vi "Teleop.vi"(10 "Match Info":T1={"Autonomous Elapsed Seconds"=0.0, "TeleOp Elapsed Seconds"=0.0, "Disabled Elapsed Seconds"=0.0, "Visited Autonomous"=FALSE, "Visited TeleOp"=FALSE, "Visited Disabled"=FALSE, "Autonomous Settings"={"Autonomous Style"=enum."Independent", "VI Refnum"=refnum}}) -> ()   [LabVIEW 2017]
doc: "This VI is called for each TeleOp packet received from the DS where the robot is not disabled. It is often used to read from the joysticks and update I/O or to update setpoints for timed control loops. It should complete and return within 20 milliseconds or it may miss DS packets."
uses:
  <vilib>/Rock Robotics/WPI/DriverStation/WPI_DriverStationMatch Info.ctl
  <vilib>/Rock Robotics/WPI/Utilities/WPI_GetSetVariantRefNum.vi
  Robot Global Data.vi
  <vilib>/Rock Robotics/Network Tables/NT Read Boolean.vi
  <vilib>/Rock Robotics/Network Tables/NT Read Number.vi
  <vilib>/Rock Robotics/Network Tables/NT Write Numeric Array.vi
panel:
  out "Sample Slider 0":dbl(slide) scale=0.0..5.0
  out "Sample Boolean 1":bool
  out "Sample Boolean 0":bool
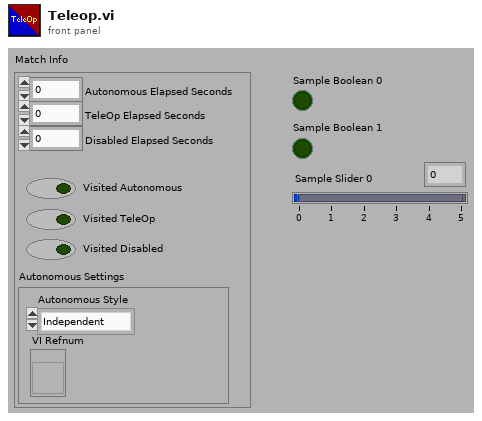
[diagram p1: front panel]
types:
  T1 = typedef "WPI_DriverStationMatch Info.ctl" = cluster{"Autonomous Elapsed Seconds":dbl, "TeleOp Elapsed Seconds":dbl, "Disabled Elapsed Seconds":dbl, "Visited Autonomous":bool, "Visited TeleOp":bool, "Visited Disabled":bool, "Autonomous Settings":cluster{"Autonomous Style":enum16{"Iterative", "Independent"}, "VI Refnum":refnum<vi>}}
  T2 = typedef "WPI_RobotDriveDevRef.ctl" = cluster{"DevStatus":errorcluster, "Motors[]":T3[], "Square Inputs":bool, "Max Output":dbl}
  T3 = typedef "WPI_MotorControlDeviceRef.ctl" = cluster{"DeviceStatus":errorcluster, "Type":T4, "PWM":cluster{"PWM Channel":T5, "DeadBand":T6}, "CAN":cluster{"Device Number":u8, "SetOutput VI Ref":variant, "GetOutput VI Ref":variant, "Enable VI Ref":variant, "Disable VI Ref":variant, "Data":variant}, "Invert":bool, "DIO PWM":cluster{"PWM \"Enable\" Channel":T5, "DIOChannel":T7, "PWM Rate":dbl}}
  T4 = typedef "WPI_MotorControlType.ctl" = enum16{"PWM", "CAN", "DIO PWM"}
  T5 = typedef "FPGA_DIOPWMChannel.ctl" = enum8{"PWM 0", "PWM 1", "PWM 2", "PWM 3", "PWM 4", "PWM 5", "PWM 6", "PWM 7", "PWM 8", "PWM 9", "PWM MXP 0", "PWM MXP 1", "PWM MXP 2", "PWM MXP 3", "PWM MXP 4", "PWM MXP 5", "PWM MXP 6", "PWM MXP 7", "PWM MXP 8", "PWM MXP 9", "Invalid"}
  T6 = typedef "WPI_PWMDeadband.ctl" = cluster{"Name":string, "maxPositivePwm":i32, "minPositivePwm":i32, "centerPwm":i32, "maxNegativePwm":i32, "minNegativePwm":i32, "angularRange":u16}
  T7 = typedef "FPGA_DIOChannel.ctl" = enum8{"DIO 0", "DIO 1", "DIO 2", "DIO 3", "DIO 4", "DIO 5", "DIO 6", "DIO 7", "DIO 8", "DIO 9", "DIO MXP 0", "DIO MXP 1", "DIO MXP 2", "DIO MXP 3", "DIO MXP 4", "DIO MXP 5", "DIO MXP 6", "DIO MXP 7", "DIO MXP 8", "DIO MXP 9", "DIO MXP 10", "DIO MXP 11", "DIO MXP 12", "DIO MXP 13", "DIO MXP 14", "DIO MXP 15", "SPI Port CS1", "SPI Port CS2", "SPI Port CS3", "SPI Port MISO", "SPI Port MOSI", "Invalid"}
  T8 = typedef "WPI_JoystickDevRef.ctl" = cluster{"Device":T9}
  T9 = typedef "WPI_JoystickDeviceEnum.ctl" = enum16{"USB 0", "USB 1", "USB 2", "USB 3", "USB 4", "USB 5"}
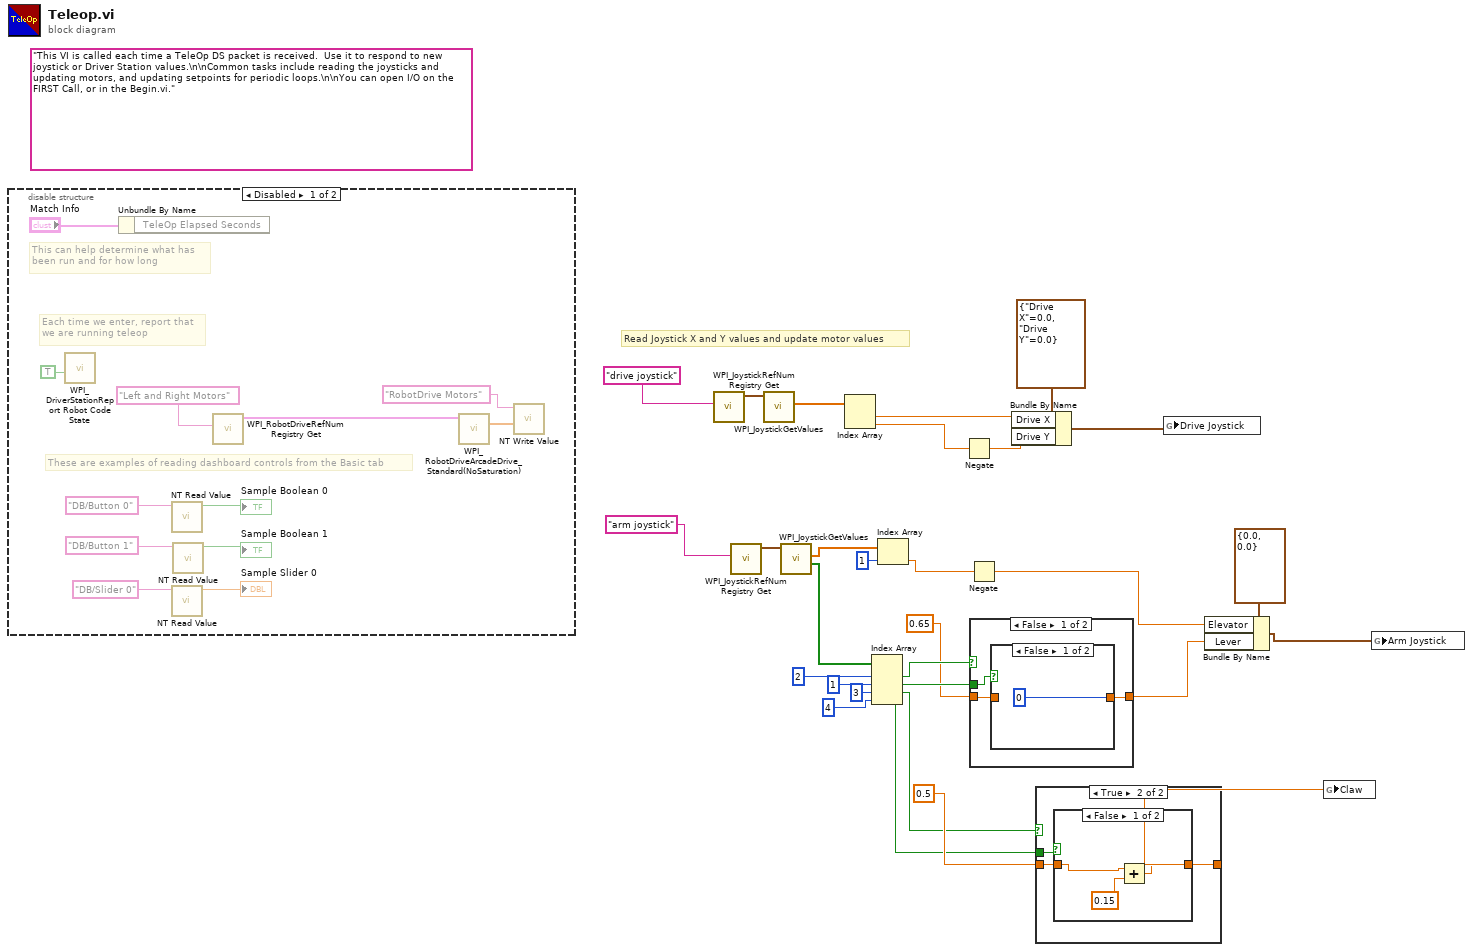
[diagram p0: block diagram]
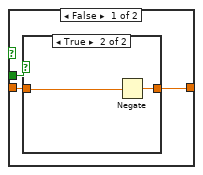
[diagram p2: hidden frame]
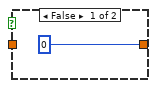
[diagram p3: hidden frame]
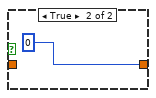
[diagram p4: hidden frame]
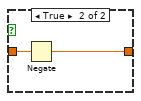
[diagram p5: hidden frame]
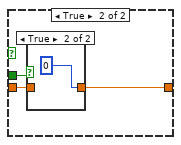
[diagram p6: hidden frame]
diagram:
  (unwired) "This VI is called each time a TeleOp DS packet is received.  Use it to respond to new joystick or Driver Station values.\n\nCommon tasks include reading the joysticks and updating motors, and updating setpoints for periodic loops.\n\nYou can open I/O on the FIRST Call, or in the Begin.vi."
  # "Read Joystick X and Y values and update motor values"
  n1 = disable-structure shown="Disabled" {
    frame Disabled {
      # "These are examples of reading dashboard controls from the Basic tab"
      # "Each time we enter, report that\nwe are running teleop"
      # "This can help determine what has\nbeen run and for how long"
      n2 = call <vilib>:"WPI_DriverStationReport Robot Code State.vi"("TeleOp"=TRUE ("Autonomous")) -> ()  [unwired: 10 in, 1 out]
      n3 = Unbundle By Name("Match Info") -> ()  [unwired: 1 out]
      n4 = call-poly <vilib>:"NT Read Value.vi"("Name"="DB/Button 0" ("refnum name")) -> ("Boolean"=→"Sample Boolean 0":bool)  [unwired: 9 in, 1 out]
      n5 = call-poly <vilib>:"NT Read Value.vi"("Name"="DB/Slider 0" ("refnum name")) -> ("Numeric"=→"Sample Slider 0":dbl)  [unwired: 9 in, 1 out]
      n6 = call-poly <vilib>:"NT Read Value.vi"("Name"="DB/Button 1" ("refnum name")) -> ("Boolean"=→"Sample Boolean 1":bool)  [unwired: 9 in, 1 out]
      n7 = call <vilib>:"WPI_RobotDriveRefNum Registry Get.vi"("refnum name"="Left and Right Motors") -> ("RobotDriveDevRef"=w32:T2)  [unwired: 1 in, 9 out]
      n8 = call <vilib>:"WPI_RobotDriveArcadeDrive_Standard(NoSaturation).vi"("RobotDriveDevRef"=w32) -> ("Motor Values"=w33:dbl[])  [unwired: 3 in, 7 out]
      n9 = call-poly <vilib>:"NT Write Value.vi"("Numeric Array"=w33, "Name"="RobotDrive Motors") -> ()  [unwired: 9 in, 1 out]
    }
    frame Enabled {
    }
  }
  n10 = call <vilib>:"WPI_JoystickRefNum Registry Get.vi"("refnum name"="drive joystick") -> ("JoystickDevRef"=w28:T8)  [unwired: 1 in, 9 out]
  n11 = call <vilib>:"WPI_JoystickRefNum Registry Get.vi"("refnum name"="arm joystick") -> ("JoystickDevRef"=w21:T8)  [unwired: 1 in, 9 out]
  n12 = call <vilib>:"WPI_JoystickGetValues.vi"("JoystickDevRef"=w28) -> ("Axes"=w27:dbl[])  [unwired: 6 in, 4 out]
  n13 = call <vilib>:"WPI_JoystickGetValues.vi"("JoystickDevRef"=w21) -> ("Buttons"=w19:bool[], "Axes"=w15:dbl[])  [unwired: 6 in, 3 out]
  n14 = Index Array(array=w27) -> (element #1=w24:dbl, element #2=w26:dbl)  [unwired: 2 in]
  n15 = Index Array(array=w19, index #1=2 ("index"), index #2=1 ("index"), index #3=3 ("index"), index #4=4 ("index")) -> (element #1=w18:bool, element #2=w17:bool, element #3=w3:bool, element #4=w2:bool)
  n16 = Index Array(array=w15, index=1) -> (element=w13:dbl)
  n17 = Negate(x=w26) -> (-x=w25:dbl)
  n18 = Negate(x=w13) -> (-x=w9:dbl)
  n19 = case shown="False" w18 {
    tunnel: w17 -> [w44 w50]
    tunnel: 0.65 -> [w43 w49]
    tunnel: [w42 w48] -> w7
    frame False {
      n20 = case shown="False" w44 {
        tunnel: w43 -> [_ w47]
        tunnel: [0 w46] -> w42
        frame False {
        }
        frame True {
          n21 = Negate(x=w47) -> (-x=w46:dbl)
        }
      }
    }
    frame True {
      n22 = case shown="True" w50 {
        tunnel: w49 -> [w51 _]
        tunnel: [w51 0] -> w48
        frame False {
        }
        frame True {
        }
      }
    }
  }
  n23 = Bundle By Name(cluster=cluster{"Drive X":dbl, "Drive Y":dbl} {"Drive X"=0.0, "Drive Y"=0.0}, "Drive X"=w24, "Drive Y"=w25) -> (w22:cluster{"Drive X":dbl, "Drive Y":dbl})
  n24 = case shown="True" w3 {
    tunnel: w2 -> [w55 w61]
    tunnel: 0.5 -> [w54 w60]
    tunnel: [w53 w59] -> w1
    frame False {
      n25 = case shown="True" w55 {
        tunnel: w54 -> [_ w57]
        tunnel: [0 w58] -> w53
        frame False {
        }
        frame True {
          n26 = Negate(x=w57) -> (-x=w58:dbl)
        }
      }
    }
    frame True {
      n27 = case shown="False" w61 {
        tunnel: w60 -> [w63 _]
        tunnel: [w62 0] -> w59
        frame False {
          n28 = Add(x=w63, y=0.15) -> (x+y=w62:dbl)
        }
        frame True {
        }
      }
    }
  }
  n29 = global write "Robot Global Data.vi" "Drive Joystick"(w22) -> ()
  n30 = Bundle By Name(cluster=cluster{"Elevator":dbl, "Lever":dbl} {"Elevator"=0.0, "Lever"=0.0} ("input cluster"), "Elevator"=w9, "Lever"=w7) -> (w6:cluster{"Elevator":dbl, "Lever":dbl})
  n31 = global write "Robot Global Data.vi" "Claw"(w1) -> ()
  n32 = global write "Robot Global Data.vi" "Arm Joystick"(w6) -> ()
